vi "Get Components.vi"(8 "error in":errorcluster, 11 "Elite DAQ Board in":refnum<class "Elite DAQ Design.lvclass">) -> (0 "error out":errorcluster, 2 "components":refnum<class "Component.lvclass">[](array[class]), 3 "Elite DAQ Board out":refnum<class "Elite DAQ Design.lvclass">)   [LabVIEW 2023, in "Elite DAQ Design.lvclass"]
doc: "Get an array of components for the board."
uses:
  Elite DAQ Design.lvclass
  Component/Component.lvclass
  MagicSignalFilter/Magic Signal Filter.lvclass
  c:/dev/_r/4/eng/lv-core/lvpostprocessingd/lv_mc_x86_64/dist_i386/examples/Object-Oriented Programming/Board Testing/Object Design/Component/Component.lvclass
  DAQBoard/DAQ Board Design.lvclass
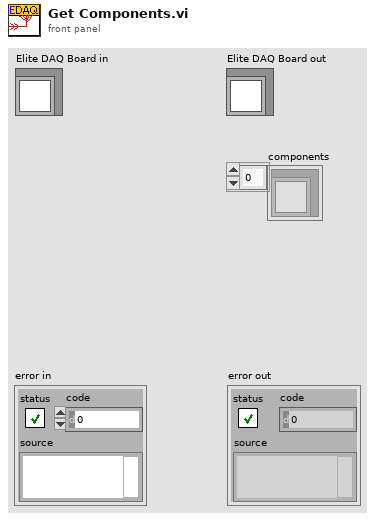
[diagram p1: front panel]
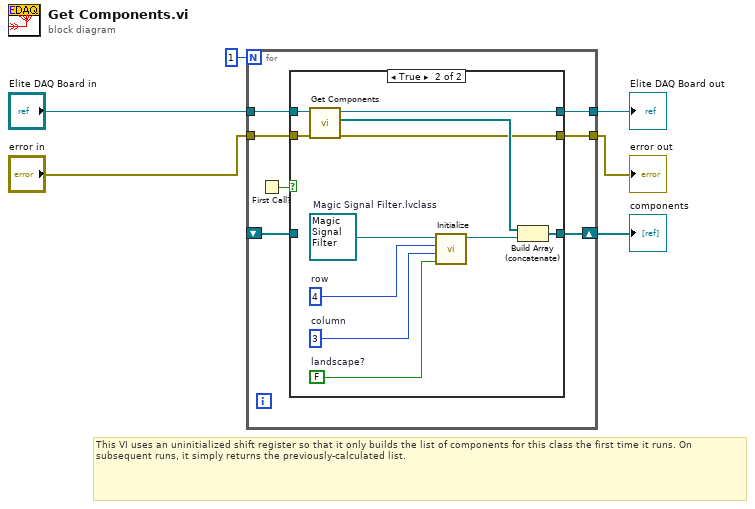
[diagram p0: block diagram]
diagram:
  # "This VI uses an uninitialized shift register so that it only builds the list of components for this class the first time it runs. On subsequent runs, it simply returns the previously-calculated list."
  n1 = for {
    N: 1 -> [_]
    tunnel: "Elite DAQ Board in" -> [w13]
    tunnel: "error in" -> [w12]
    tunnel: [w11] -> w4
    tunnel: [w10] -> w3
    shift-right: [w9] -> w2
    shift-left: _ -> [w7]
    n2 = First Call?() -> (First Call?: T/F=w8:bool)
    n3 = case shown="True" w8 {
      tunnel: w13 -> [w16 w27]
      tunnel: w12 -> [w15 w26]
      tunnel: [w16 w24] -> w11
      tunnel: [w15 w23] -> w10
      tunnel: [w14 w22] -> w9
      tunnel: w7 -> [w14 _]
      frame False {
      }
      frame True {
        w19 = i16 4  # row
        w18 = i16 3  # column
        w17 = FALSE  # landscape?
        w21 = refnum<class "Magic Signal Filter.lvclass"> refnum  # Magic Signal Filter.lvclass
        n4 = call-parent "Get Components.vi"("error in"=w26, "DAQ Board in"=w27) -> ("error out"=w23:errorcluster, "components"=w25:refnum<class "Component.lvclass">[], "DAQ Board out"=w24:refnum<class "Elite DAQ Design.lvclass">)  [unwired: 7 in]
        n5 = call "Initialize.vi"("landscape?"=w17, "column"=w18, "row"=w19, "Component.lvclass in"=w21) -> ("Component.lvclass out"=w20:refnum<class "Magic Signal Filter.lvclass">)  [unwired: 7 in]
        n6 = Build Array (concatenate)(w25, w20) -> (w22:refnum<class "Component.lvclass">[])
      }
    }
  }
  "error out" <- w3
  "Elite DAQ Board out" <- w4
  "components" <- w2
